vi "DevB.Get Data.vi"   [LabVIEW 2018]
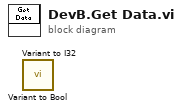
[diagram p0: block diagram]
diagram:
  n1 = call "Variant to Bool.vi"() -> ()  [unwired: 10 in, 2 out]
  n2 = call "Variant to I32.vi"() -> ()  [unwired: 10 in, 2 out]
